vi "Untitled 1.vi"() -> ()   [LabVIEW 2019]
uses:
  examples/route_guide/route_guide_client/RPC Messages/routeguide_RouteNote.ctl
  examples/route_guide/route_guide_client/RPC Messages/routeguide_Point.ctl
  <vilib>/gRPC/LabVIEW gRPC Library/grpc-lvsupport-release.lvlib
  Generated_client/Generated_client.lvlib
  examples/route_guide/route_guide_client/route_guide_client.lvlib
panel:
  in  "error in":errorcluster
  out "error out":errorcluster
  out "Response Data":T1[](array[typedef])
  in  "Request Data":T1[](array[typedef])=[{"location"={"latitude"=1, "longitude"=1}, "message"="Point 1"}, {"location"={"latitude"=2, "longitude"=2}, "message"="Point 2"}]
  in  "Server Address":string="localhost:50051"
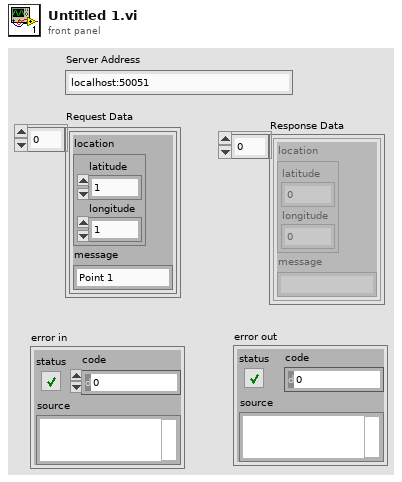
[diagram p1: front panel]
types:
  T1 = typedef "route_guide_client.lvlib/routeguide_RouteNote.ctl" = cluster{"location":T2, "message":string}
  T2 = typedef "route_guide_client.lvlib/routeguide_Point.ctl" = cluster{"latitude":i32, "longitude":i32}
  T3 = typedef "grpc-lvsupport-release.lvlib/grpcId.ctl" = u64
  T4 = typedef "Generated_client.lvlib/routeguide_RouteNote.ctl" = cluster{"location":T5, "message":string}
  T5 = typedef "Generated_client.lvlib/routeguide_Point.ctl" = cluster{"latitude":i32, "longitude":i32}
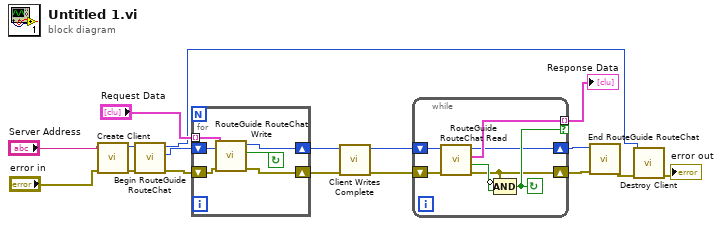
[diagram p0: block diagram]
diagram:
  n1 = call "Create Client.vi"("error in"="error in", "address"="Server Address") -> ("error out"=w8:errorcluster, "gRPC ID Out"=w9:T3)  [unwired: 8 in]
  n2 = call "Begin RouteGuide RouteChat.vi"("error in"=w8, "gRPC ID"=w9) -> ("error out"=w7:errorcluster, "Call Id Out"=w6:T3, "gRPC ID out"=w3:T3)  [unwired: 7 in]
  n3 = for {
    shift-right: [w20] -> w15
    shift-left: w6 -> [w23]
    shift-right: [w21] -> w13
    shift-left: w7 -> [w22]
    tunnel: "Request Data" -> [w18] mode=indexing
    stop <- w19 continue-if-true
    n4 = call "RouteGuide RouteChat Write.vi"("error in"=w22, "Request Data"=w18, "Call ID in"=w23) -> ("error out"=w21:errorcluster, "Success"=w19:bool, "Call ID"=w20:T3)  [unwired: 6 in]
  }
  n5 = call <vilib>:"Client Writes Complete.vi"("error in"=w13, "ClientID in"=w15) -> ("error out"=w12:errorcluster, "ClientID out"=w14:T3)  [unwired: 8 in]
  n6 = while {
    shift-right: [w26] -> w5
    shift-left: w14 -> [w29]
    shift-right: [w24] -> w4
    shift-left: w12 -> [w28]
    tunnel: [w27] -> w16 mode=indexing if=w30
    stop <- w30 continue-if-true
    n7 = call "RouteGuide RouteChat Read.vi"("error in"=w28, "Call ID in"=w29) -> ("error out"=w24:errorcluster, "Success"=w25:bool, "Response Data"=w27:T4, "Call ID"=w26:T3)  [unwired: 6 in]
    n8 = Compound Arithmetic op=AND(invert w24, w25) -> (w30:bool)
  }
  "Response Data" <- w16
  n9 = call "End RouteGuide RouteChat.vi"("error in"=w4, "Call ID in"=w5) -> ("error out"=w1:errorcluster)  [unwired: 8 in, 1 out]
  n10 = call "Destroy Client.vi"("error in"=w1, "gRPC ID"=w3) -> ("error out"=→"error out":errorcluster)  [unwired: 9 in]
